vi "CO Gas Preparation.vi"() -> ()   [LabVIEW 2014]
panel:
  out "CO preflight Des 1":string="CO Ground Preflight Checks - DO NOT GET DISTRACTED!\n\n1. COCYL1\n    Open Manual Valve V1 (anticlockwise)\n    Note down ALREG1 content bar pressure in e-Log (bottom gauge)    \n    Check ALREG1 delivery pressure > 2 bar (top gauge)\n    Open Green Manual Valve V2\n\n2. COCYL2\n    Open Manual Valve V3 (anticlockwise)\n    Note down ALREG2 content bar pressure in e-Log (bottom gauge) \n    Check ALREG2 delivery pressure > 2 bar (top gauge)\n    Open Green Manual Valves V4 and V5\n\n3. COCYL3 - Purging CO/Air cal gas\n\n\n\n\n\n\n\n\n\n\n\n\n\na) Disconnect quick connector from \"Instrument\"\nb) Connect to \"Purge\" quick connector\nc) Wait for pressure regulator ALREG3 top and bottom gauges to drop to zero\nd) Back out ALREG3 delivery pressure control valve\ne) Open / Close COCYL3 (V8) cylinder valve\nf) Increase delivery pressure to purge regulator (clockwise)\ng) Wait for pressure regulator ALREG3 top & bottom gauges to drop to zero\nh) Repeat steps d) to g) three more times\n\ni) Back out ALREG3 delivery pressure control valve (fully counter clockwise)\n\nj) Connect to \"Instrument\" quick connector (THIS IS A CRITICAL STEP!)\n\nk) Open COCYL3 (V8)\nl) Set ALREG3 delivery pressure control valve to 3 bar"
  in  "Exit":bool
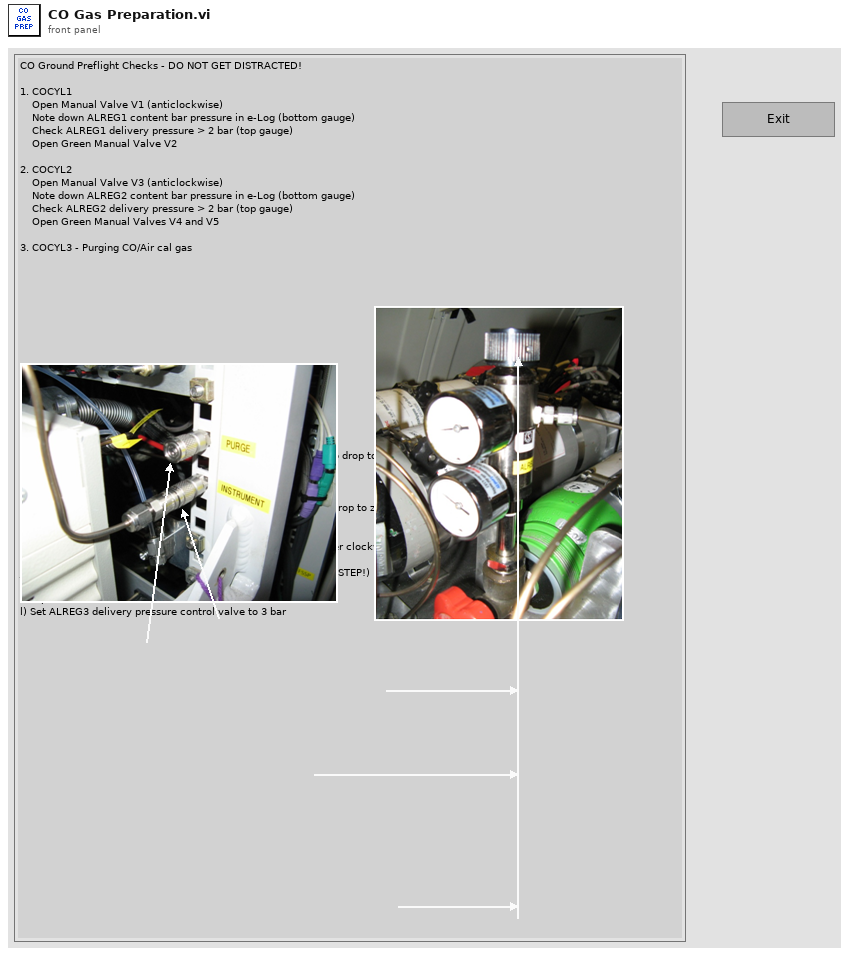
[diagram p1: front panel]
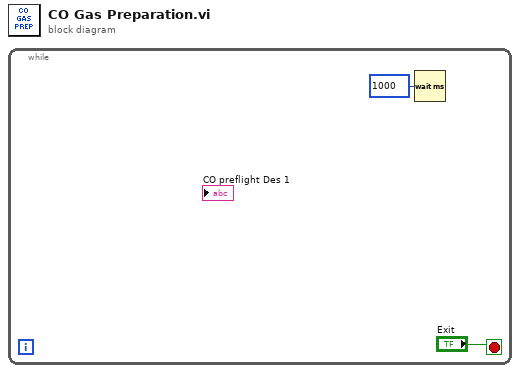
[diagram p0: block diagram]
diagram:
  n1 = while {
    stop <- "Exit" stop-if-true
    n2 = Wait (ms)(milliseconds to wait=u32 1000) -> ()  [unwired: 1 out]
  }
